vi "UBX Checksum.vi"(8 "error in":errorcluster, 10 "Checksum Packet":i8[](array[numeric]) format="%x", 11 "VISA resource name":refnum<visa-resource-name>) -> (0 "error out":errorcluster, 1 "CK_B":i8, 2 "CK_A":i8, 3 "VISA resource name out":refnum<visa-resource-name>)   [LabVIEW 2011, in "u-blox 5 Series.lvlib"]
doc: "Calculates a Fletcher's Checksum over the packet. See the UBX Protocol Specifications for more details."
uses:
  u-blox 5 Series.lvlib
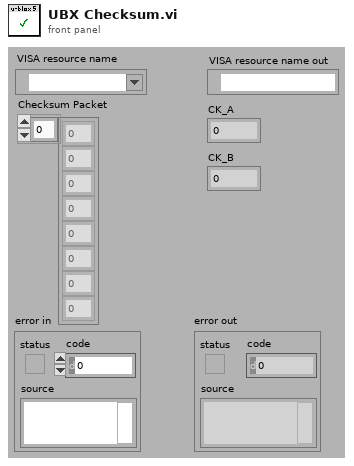
[diagram p1: front panel]
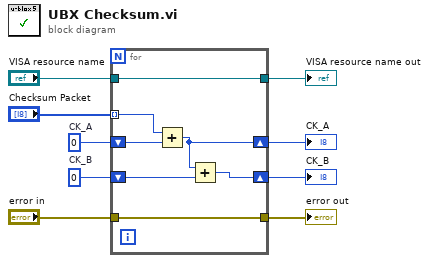
[diagram p0: block diagram]
diagram:
  w9 = i8 0  # CK_B
  w8 = i8 0  # CK_A
  n1 = for {
    shift-right: [w15] -> w5
    shift-left: w9 -> [w16]
    shift-right: [w10] -> w6
    shift-left: w8 -> [w14]
    tunnel: "Checksum Packet" -> [w13] mode=indexing
    tunnel: "error in" -> [w12]
    tunnel: [w12] -> w3
    tunnel: "VISA resource name" -> [w11]
    tunnel: [w11] -> w1
    n2 = Add(x=w13, y=w14) -> (x+y=w10:i8)
    n3 = Add(x=w10, y=w16) -> (x+y=w15:i8)
  }
  "VISA resource name out" <- w1
  "error out" <- w3
  "CK_A" <- w6
  "CK_B" <- w5
